vi "Configure Modulation (Frequency-Shift Keying).vi"(0 "VISA resource name":refnum<visa-resource-name>, 1 "FSK Source (0: Internal)":i32(ring) items=["Internal", "External", "CH1", "CH2"], 5 "Channel (1: 1)":i32(ring)=1 items=["1"=1, "2"=2], 7 "Enable FSK Modulation(T: Enable)":bool=TRUE, 11 "error in (no error)":errorcluster, 12 "FSK Alternate Frequency (100 Hz)":dbl=100.0, 13 "FSK Rate (100 Hz)":dbl=100.0) -> (4 "VISA resource name out":refnum<visa-resource-name>, 15 "error out":errorcluster)   [LabVIEW 2020, in "AWG.lvlib" / "Agilent 3352X Series.lvlib"]
doc: "Allows and configures Frequency-Shift Keying (FSK) modulation. The function generator shifts its output frequency between two present values. The carrier waveform shape and parameters are set by config waveform function.\n\n<b>Note</b>:\n(1) When enabling this mode, all other modes will be turned off.\n(2) The carrier waveform shape and parameters are set by the Configure Standard Waveform vi. You can select a sine, square, ramp, or pulse waveform for the carrier (arbitrary, noise, PRBS, and DC are not allowed). \n(3) Use Configure Pulse Waveform VI to select Pulse shape and set the parameters"
uses:
  Agilent 3352X Series.lvlib
panel:
  # "Internal FSK Modulation Settings"
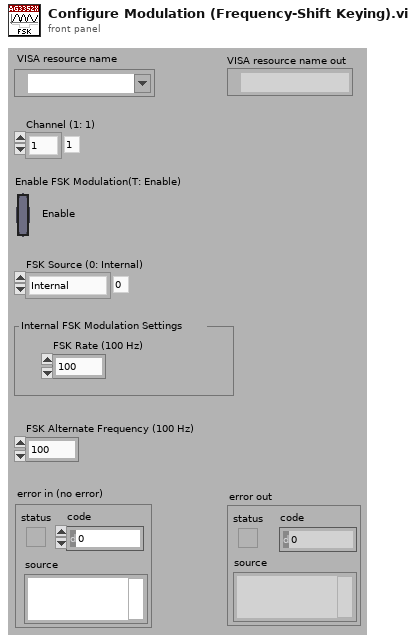
[diagram p1: front panel]
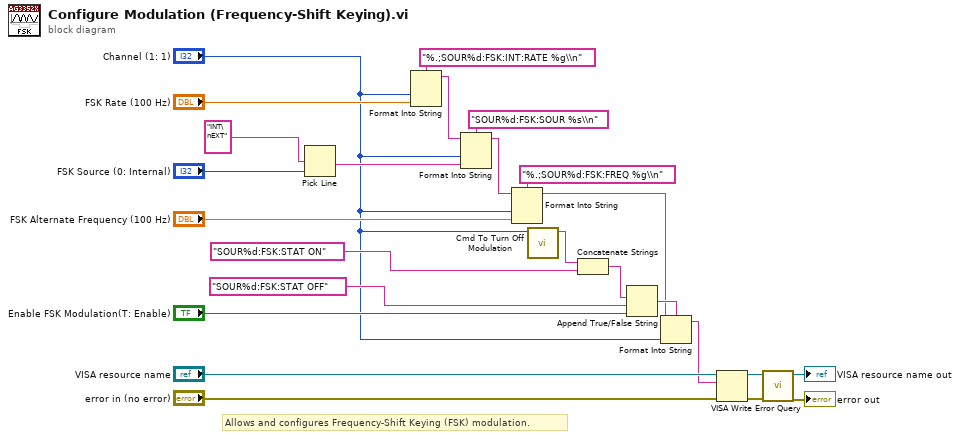
[diagram p0: block diagram]
diagram:
  # "Allows and configures Frequency-Shift Keying (FSK) modulation."
  n1 = Pick Line(multi-line string="INT\nEXT", line index="FSK Source (0: Internal)") -> (output string=w11:string)  [unwired: 1 out]
  n2 = Format Into String(format string="%.;SOUR%d:FSK:INT:RATE %g\\n", "Channel (1: 1)", "FSK Rate (100 Hz)") -> (resulting string=w23:string)  [unwired: 2 in, 1 out]
  n3 = Format Into String(format string="SOUR%d:FSK:SOUR %s\\n", initial string=w23, "Channel (1: 1)", w11) -> (resulting string=w5:string)  [unwired: 1 in, 1 out]
  n4 = Format Into String(format string="%.;SOUR%d:FSK:FREQ %g\\n", initial string=w5, "Channel (1: 1)", "FSK Alternate Frequency (100 Hz)") -> (resulting string=w2:string)  [unwired: 1 in, 1 out]
  n5 = call "Cmd To Turn Off Modulation.vi"("Channel (1: 1)"="Channel (1: 1)") -> ("Cmd String"=w7:string)  [unwired: 10 out]
  n6 = Concatenate Strings(w7, "SOUR%d:FSK:STAT ON") -> (w10:string)
  n7 = Append True/False String(1:"Enable FSK Modulation(T: Enable)", 2:"SOUR%d:FSK:STAT OFF", 3:w10) -> (0:w9:string)  [unwired: 1 out]
  n8 = Format Into String(format string=w9, initial string=w2, "Channel (1: 1)") -> (resulting string=w1:string)  [unwired: 1 in, 1 out]
  n9 = VISA Write(VISA resource name="VISA resource name", write buffer=w1, error in (no error)="error in (no error)") -> (VISA resource name out=w17:refnum<visa-resource-name>, error out=w16:errorcluster)  [unwired: 1 out]
  n10 = call "Error Query.vi"("error in (no error)"=w16, "VISA resource name"=w17) -> ("error out"=→"error out":errorcluster, "VISA resource name out"=→"VISA resource name out":refnum<visa-resource-name>)  [unwired: 8 out]
